vi "Set Single Track.vi"(10 "height":i32, 11 "centre":i32) -> (3 "function return":u32)   [LabVIEW 2018, in "AndorSDK.lvlib"]
doc: "EXPNETTYPE unsigned int WINAPI SetSingleTrack(int centre, int height);"
uses:
  AndorSDK.lvlib
  ATMCD32D.dll
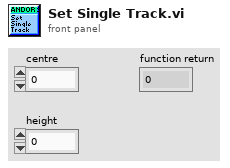
[diagram p1: front panel]
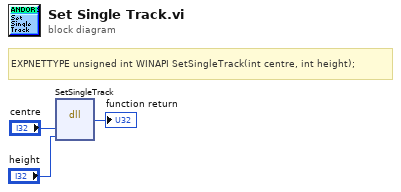
[diagram p0: block diagram]
diagram:
  # "EXPNETTYPE unsigned int WINAPI SetSingleTrack(int centre, int height);"
  n1 = dll-call lib="PTH2babs E\nPersönliches02 - Arbeit03-HiwijobsLabviewCodelibANDOR\tAndor SDK\nATMCD32D.*" fn="SetSingleTrack"("centre"="centre", "height"="height") -> (→"function return":u32)  [unwired: 5 in, 2 out]
